vi "AG33XXX.get interface.vi"(0 "i ref in":refnum<vi>, 5 "error in (no error)":errorcluster) -> (14 "i ref out":refnum<vi>, 16 "interface":refnum<visa-resource-name>, 19 "error out":errorcluster)   [LabVIEW 2014, in "AG33XXX.lvlib"]
doc: "Gets the VISA string from the BaseProcess i attributes. That string is needed when calling the instrument driver within the methods of this class."
uses:
  AG33XXX.lvlib
  CSCore/BaseProcess/BaseProcess.lvlib
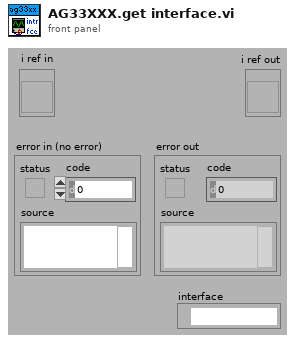
[diagram p1: front panel]
types:
  T1 = typedef "BaseProcess.lvlib/BaseProcess.i attribute.ctl" = cluster{"EventStatus":string, "EventError":i32, "PresetEvtWatchD":i32, "PresetPdcWatchD":i32, "EventTimeout":i32, "PeriodicInterval":i32, "Interface":string[], "Address":string[], "Special":string[], "PeriodicError":i32, "PeriodicStatus":string, "SuperProc":string, "Descriptors":T2[], "CaseRef":refnum<vi>, "PdcRef":refnum<vi>, "Thread Ref":refnum<vi>, "eventErrorID":i32, "eventStatusID":i32, "periodicErrorID":i32, "periodicStatusID":i32, "pdcCtrID":i32}
  T2 = typedef "BaseProcess.lvlib/BaseProcess.descriptor definition.ctl" = cluster{"selector":string, "descriptor":T3}
  T3 = typedef "BaseProcess.lvlib/BaseProcess.descriptor string definition.ctl" = string
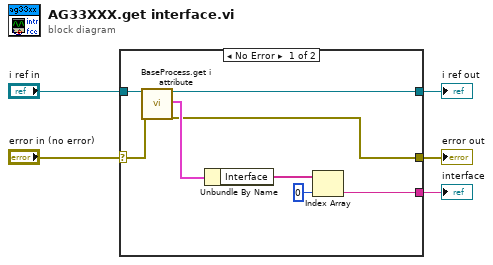
[diagram p0: block diagram]
diagram:
  n1 = case shown="No Error" "error in (no error)" {
    selector: "error in (no error)" -> [w7 w14]
    tunnel: "i ref in" -> [w13 w15]
    tunnel: [w6 _] -> w4
    tunnel: [w9 w15] -> w3
    tunnel: [w8 w14] -> w2
    frame No Error {
      n2 = call "BaseProcess.get i attribute.vi"("i ref in"=w13, "error in (no error)"=w7) -> ("i ref out"=w9:refnum<vi>, "i attribute"=w10:T1, "error out"=w8:errorcluster)  [unwired: 15 in]
      n3 = Unbundle By Name(w10) -> ("Interface"=w12:string[])
      n4 = Index Array(array=w12, index=0 ("Index")) -> (element=w6:string)
    }
    frame Error {
    }
  }
  "error out" <- w2
  "i ref out" <- w3
  "interface" <- w4
